vi "lv class tree.vi"() -> ()   [LabVIEW 2012]
uses:
  <vilib>/_script/All Supported PropertiesOrMethods TypeDefs/ASC_ArrayOfUniqueIDStringParentIDStringName.ctl
  <vilib>/_script/All Supported PropertiesOrMethods TypeDefs/ASC_UniqueIDStringParentIDStringName.ctl
panel:
  out "parent_children":cluster{i32[], string[], i32[], string[]}[](array[cluster])
  out "children":T1(array[cluster])
  out "sorted array 2":cluster{i32[], string[]}[](array[cluster])
  out "element 3":T2
  in  "element":string
  out "sorted array":T3(array[cluster])
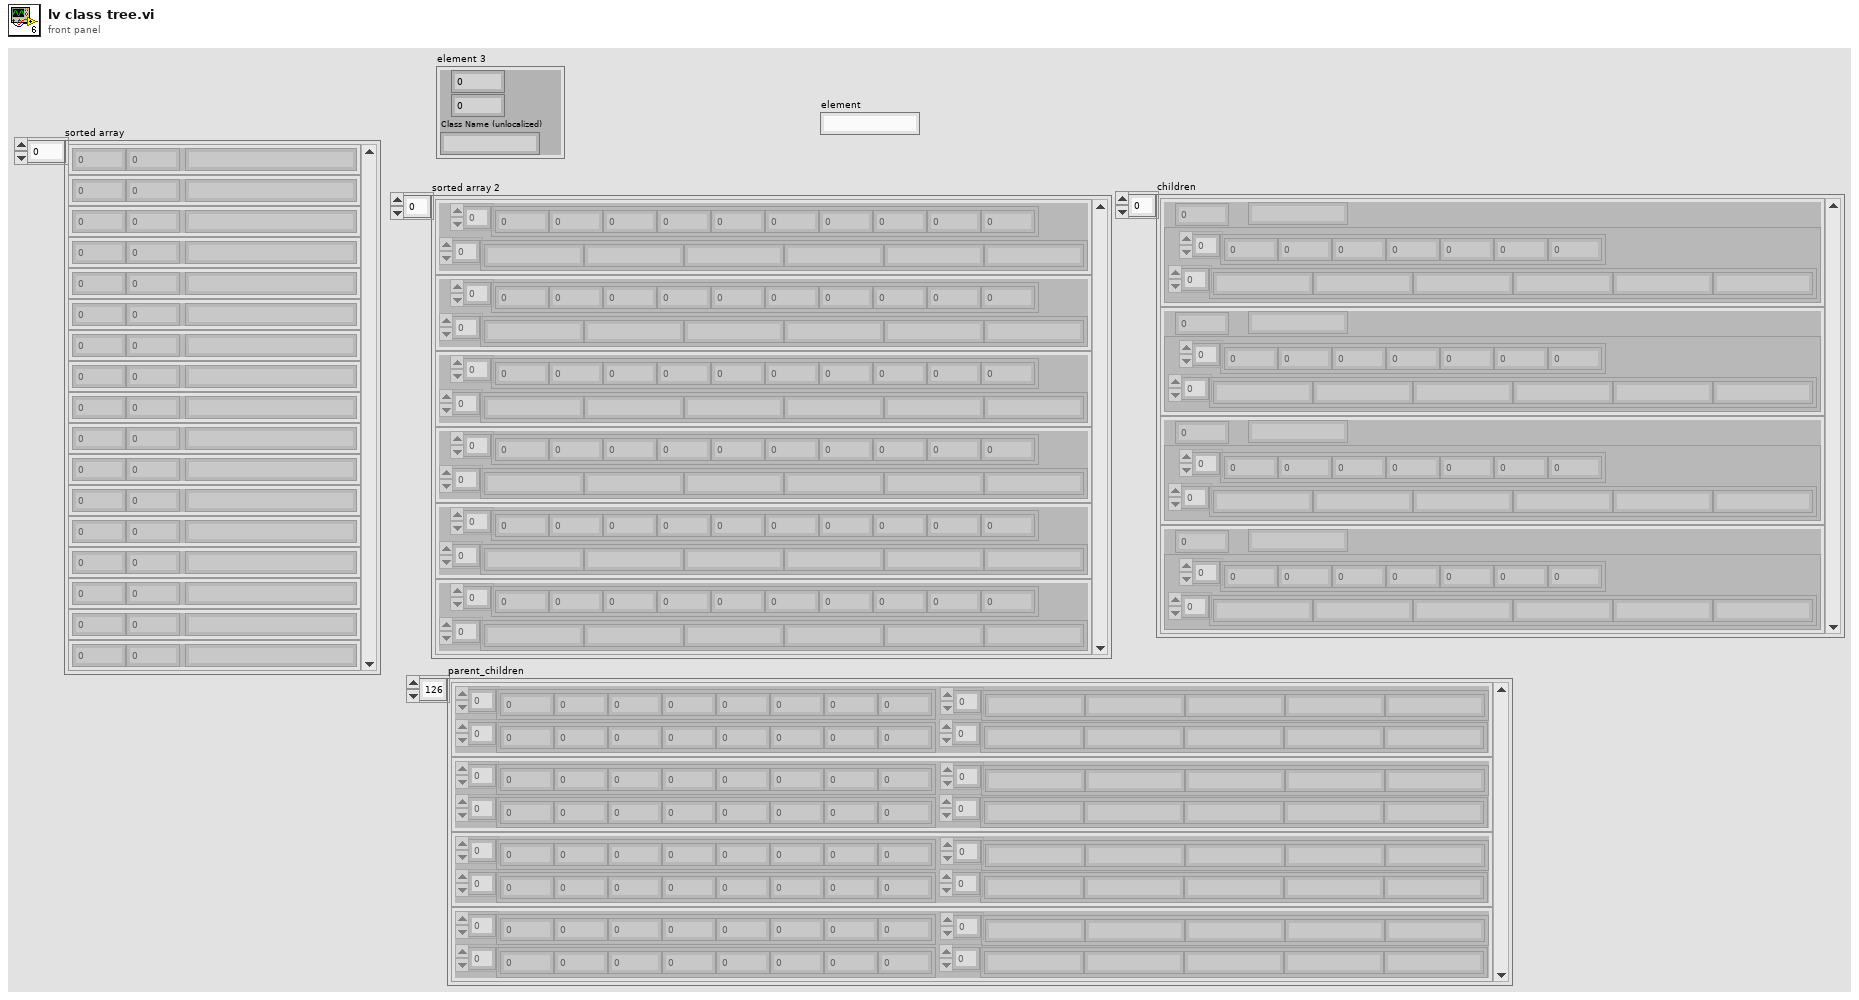
[diagram p1: front panel]
types:
  T1 = cluster{i32, cluster{i32[], string[]}, "Class Name (unlocalized)":string}[]
  T2 = cluster{i32, i32, "Class Name (unlocalized)":string}
  T3 = cluster{i32, i32, "Class Name (unlocalized)":string}[]
  T4 = typedef "ASC_ArrayOfUniqueIDStringParentIDStringName.ctl" = T5[]
  T5 = typedef "ASC_UniqueIDStringParentIDStringName.ctl" = cluster{"Unique ID string":string, "Parent ID string":string, "Class Name (unlocalized)":string, "Class Name (localized)":string}
  T6 = cluster{"Class Name (unlocalized)":string, i32, i32}
  T7 = cluster{"Class Name (unlocalized)":string, i32, i32}[]
  T8 = cluster{i32, cluster{i32[], string[]}, "Class Name (unlocalized)":string}
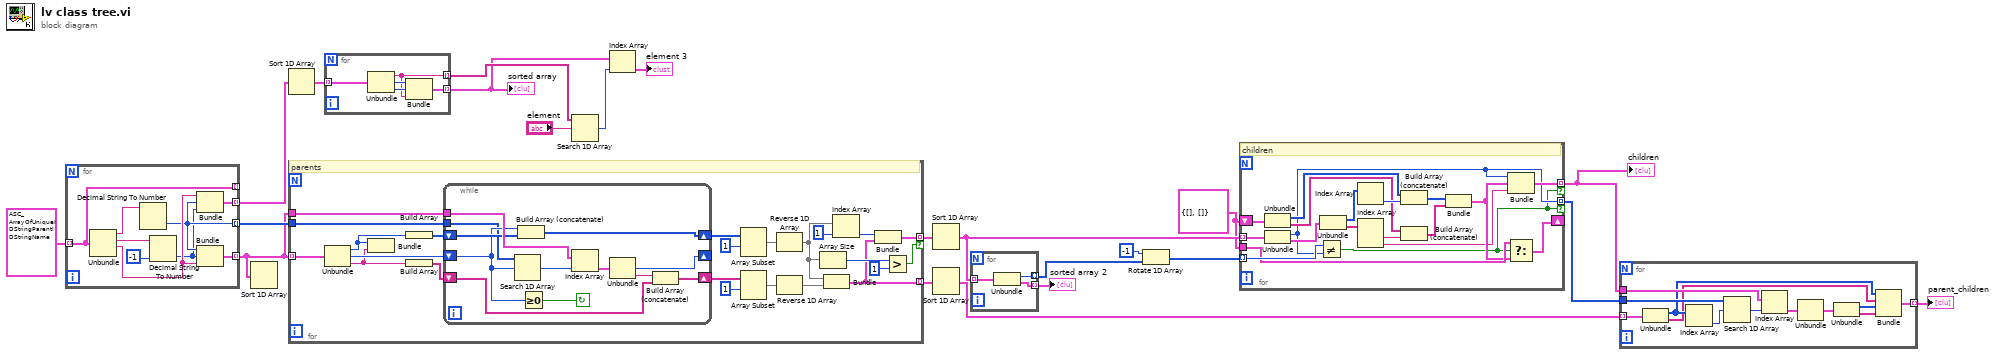
[diagram p0: block diagram]
diagram:
  w6 = cluster{i32[], string[]} {[], []} ("output cluster")
  n1 = for {
    tunnel: [w27] -> _ mode=indexing
    tunnel: [w28] -> w19 mode=indexing
    tunnel: [w25] -> w22 mode=indexing
    tunnel: T4 [{"Unique ID string"="3", "Parent ID string"="", "Class Name (unlocalized)"="Generic", "Class Name (localized)"="Generic"}, {"Unique ID string"="1", "Parent ID string"="", "Class Name (unlocalized)"="Application", "Class Name (localized)"="Application"}, {"Unique ID string"="2", "Parent ID string"="", "Class Name (unlocalized)"="VI", "Class Name (localized)"="VI"}, {"Unique ID string"="73", "Parent ID string"="", "Class Name (unlocalized)"="Project", "Class Name (localized)"="Project"}, {"Unique ID string"="74", "Parent ID string"="", "Class Name (unlocalized)"="ProjectItem", "Class Name (localized)"="ProjectItem"}, {"Unique ID string"="101", "Parent ID string"="2", "Class Name (unlocalized)"="PolymorphicVI", "Class Name (localized)"="PolymorphicVI"}, {"Unique ID string"="79", "Parent ID string"="2", "Class Name (unlocalized)"="FacadeVI", "Class Name (localized)"="FacadeVI"}, {"Unique ID string"="80", "Parent ID string"="74", "Class Name (unlocalized)"="Library", "Class Name (localized)"="Library"}, {"Unique ID string"="81", "Parent ID string"="", "Class Name (unlocalized)"="Variable", "Class Name (localized)"="Variable"}, {"Unique ID string"="82", "Parent ID string"="", "Class Name (unlocalized)"="TagSet", "Class Name (localized)"="TagSet"}, {"Unique ID string"="87", "Parent ID string"="2", "Class Name (unlocalized)"="MethodVI", "Class Name (localized)"="MethodVI"}, {"Unique ID string"="103", "Parent ID string"="80", "Class Name (unlocalized)"="XInterfaceLibrary", "Class Name (localized)"="XInterfaceLibrary"}, {"Unique ID string"="88", "Parent ID string"="103", "Class Name (unlocalized)"="XControlLibrary", "Class Name (localized)"="XControlLibrary"}, {"Unique ID string"="91", "Parent ID string"="", "Class Name (unlocalized)"="LVTarget", "Class Name (localized)"="LVTarget"}, {"Unique ID string"="93", "Parent ID string"="", "Class Name (unlocalized)"="Provider", "Class Name (localized)"="Provider"}, {"Unique ID string"="94", "Parent ID string"="", "Class Name (unlocalized)"="CopyOperation", "Class Name (localized)"="CopyOperation"}, {"Unique ID string"="95", "Parent ID string"="74", "Class Name (unlocalized)"="TargetItem", "Class Name (localized)"="TargetItem"}, {"Unique ID string"="96", "Parent ID string"="", "Class Name (unlocalized)"="ProjectItemType", "Class Name (localized)"="ProjectItemType"}, {"Unique ID string"="97", "Parent ID string"="", "Class Name (unlocalized)"="CopyItem", "Class Name (localized)"="CopyItem"}, {"Unique ID string"="98", "Parent ID string"="", "Class Name (unlocalized)"="CopyConflict", "Class Name (localized)"="CopyConflict"}, {"Unique ID string"="99", "Parent ID string"="", "Class Name (unlocalized)"="CopyExpert", "Class Name (localized)"="CopyExpert"}, {"Unique ID string"="123", "Parent ID string"="", "Class Name (unlocalized)"="Scene", "Class Name (localized)"="Scene"}, {"Unique ID string"="111", "Parent ID string"="123", "Class Name (unlocalized)"="SceneTexture", "Class Name (localized)"="SceneTexture"}, {"Unique ID string"="104", "Parent ID string"="123", "Class Name (unlocalized)"="SceneNode", "Class Name (localized)"="SceneNode"}, {"Unique ID string"="106", "Parent ID string"="104", "Class Name (unlocalized)"="SceneLight", "Class Name (localized)"="SceneLight"}, {"Unique ID string"="128", "Parent ID string"="123", "Class Name (unlocalized)"="SceneDrawable", "Class Name (localized)"="SceneDrawable"}, {"Unique ID string"="112", "Parent ID string"="128", "Class Name (unlocalized)"="SceneGeometry", "Class Name (localized)"="SceneGeometry"}, {"Unique ID string"="118", "Parent ID string"="112", "Class Name (unlocalized)"="SceneMesh", "Class Name (localized)"="SceneMesh"}, {"Unique ID string"="116", "Parent ID string"="112", "Class Name (unlocalized)"="SceneHeightField", "Class Name (localized)"="SceneHeightField"}, {"Unique ID string"="115", "Parent ID string"="112", "Class Name (unlocalized)"="SceneCylinder", "Class Name (localized)"="SceneCylinder"}, {"Unique ID string"="117", "Parent ID string"="112", "Class Name (unlocalized)"="SceneSphere", "Class Name (localized)"="SceneSphere"}, {"Unique ID string"="114", "Parent ID string"="112", "Class Name (unlocalized)"="SceneCone", "Class Name (localized)"="SceneCone"}, {"Unique ID string"="113", "Parent ID string"="112", "Class Name (unlocalized)"="SceneBox", "Class Name (localized)"="SceneBox"}, {"Unique ID string"="105", "Parent ID string"="104", "Class Name (unlocalized)"="SceneObject", "Class Name (localized)"="SceneObject"}, {"Unique ID string"="110", "Parent ID string"="104", "Class Name (unlocalized)"="SceneClipPlane", "Class Name (localized)"="SceneClipPlane"}, {"Unique ID string"="84", "Parent ID string"="123", "Class Name (unlocalized)"="SceneWindow", "Class Name (localized)"="SceneWindow"}, {"Unique ID string"="120", "Parent ID string"="74", "Class Name (unlocalized)"="PropertyFolder", "Class Name (localized)"="PropertyFolder"}, {"Unique ID string"="119", "Parent ID string"="120", "Class Name (unlocalized)"="XPropertyFolder", "Class Name (localized)"="XPropertyFolder"}, {"Unique ID string"="125", "Parent ID string"="74", "Class Name (unlocalized)"="LibraryData", "Class Name (localized)"="LibraryData"}, {"Unique ID string"="129", "Parent ID string"="128", "Class Name (unlocalized)"="SceneText", "Class Name (localized)"="SceneText"}, {"Unique ID string"="62", "Parent ID string"="2", "Class Name (unlocalized)"="SubsystemVI", "Class Name (localized)"="SubsystemVI"}, {"Unique ID string"="133", "Parent ID string"="", "Class Name (unlocalized)"="ProjectFilesViewItem", "Class Name (localized)"="ProjectFilesViewItem"}, {"Unique ID string"="134", "Parent ID string"="74", "Class Name (unlocalized)"="LVClassPropDefFolder", "Class Name (localized)"="LVClassPropDefFolder"}, {"Unique ID string"="36", "Parent ID string"="3", "Class Name (unlocalized)"="GObject", "Class Name (localized)"="GObject"}, {"Unique ID string"="37", "Parent ID string"="3", "Class Name (unlocalized)"="Plot", "Class Name (localized)"="Plot"}, {"Unique ID string"="38", "Parent ID string"="3", "Class Name (unlocalized)"="Cursor", "Class Name (localized)"="Cursor"}, {"Unique ID string"="4", "Parent ID string"="36", "Class Name (unlocalized)"="Decoration", "Class Name (localized)"="Decoration"}, {"Unique ID string"="5", "Parent ID string"="4", "Class Name (unlocalized)"="Text", "Class Name (localized)"="Text"}, {"Unique ID string"="39", "Parent ID string"="5", "Class Name (unlocalized)"="NumericText", "Class Name (localized)"="NumericText"}, {"Unique ID string"="40", "Parent ID string"="36", "Class Name (unlocalized)"="Scale", "Class Name (localized)"="Scale"}, {"Unique ID string"="41", "Parent ID string"="40", "Class Name (unlocalized)"="ColorScale", "Class Name (localized)"="ColorScale"}, {"Unique ID string"="42", "Parent ID string"="40", "Class Name (unlocalized)"="GraphScale", "Class Name (localized)"="GraphScale"}, {"Unique ID string"="43", "Parent ID string"="40", "Class Name (unlocalized)"="ColorGraphScale", "Class Name (localized)"="ColorGraphScale"}, {"Unique ID string"="6", "Parent ID string"="36", "Class Name (unlocalized)"="Control", "Class Name (localized)"="Control"}, {"Unique ID string"="7", "Parent ID string"="6", "Class Name (unlocalized)"="ColorBox", "Class Name (localized)"="ColorBox"}, {"Unique ID string"="8", "Parent ID string"="6", "Class Name (unlocalized)"="Boolean", "Class Name (localized)"="Boolean"}, {"Unique ID string"="9", "Parent ID string"="6", "Class Name (unlocalized)"="RefNum", "Class Name (localized)"="RefNum"}, {"Unique ID string"="44", "Parent ID string"="9", "Class Name (unlocalized)"="TypedRefNum", "Class Name (localized)"="TypedRefNum"}, {"Unique ID string"="10", "Parent ID string"="6", "Class Name (unlocalized)"="LVVariant", "Class Name (localized)"="LVVariant"}, {"Unique ID string"="11", "Parent ID string"="6", "Class Name (unlocalized)"="Path", "Class Name (localized)"="Path"}, {"Unique ID string"="12", "Parent ID string"="6", "Class Name (unlocalized)"="ListBox", "Class Name (localized)"="ListBox"}, {"Unique ID string"="13", "Parent ID string"="6", "Class Name (unlocalized)"="Table", "Class Name (localized)"="Table"}, {"Unique ID string"="14", "Parent ID string"="6", "Class Name (unlocalized)"="Array", "Class Name (localized)"="Array"}, {"Unique ID string"="15", "Parent ID string"="6", "Class Name (unlocalized)"="Picture", "Class Name (localized)"="Picture"}, {"Unique ID string"="16", "Parent ID string"="6", "Class Name (unlocalized)"="ActiveXContainer", "Class Name (localized)"="ActiveXContainer"}, {"Unique ID string"="17", "Parent ID string"="6", "Class Name (unlocalized)"="Numeric", "Class Name (localized)"="Numeric"}, {"Unique ID string"="18", "Parent ID string"="17", "Class Name (unlocalized)"="Digital", "Class Name (localized)"="Digital"}, {"Unique ID string"="19", "Parent ID string"="17", "Class Name (unlocalized)"="NamedNumeric", "Class Name (localized)"="NamedNumeric"}, {"Unique ID string"="35", "Parent ID string"="19", "Class Name (unlocalized)"="Enum", "Class Name (localized)"="Enum"}, {"Unique ID string"="34", "Parent ID string"="19", "Class Name (unlocalized)"="Ring", "Class Name (localized)"="Ring"}, {"Unique ID string"="20", "Parent ID string"="17", "Class Name (unlocalized)"="ColorRamp", "Class Name (localized)"="ColorRamp"}, {"Unique ID string"="33", "Parent ID string"="17", "Class Name (unlocalized)"="NumericWithScale", "Class Name (localized)"="NumericWithScale"}, {"Unique ID string"="21", "Parent ID string"="33", "Class Name (unlocalized)"="Slide", "Class Name (localized)"="Slide"}, {"Unique ID string"="32", "Parent ID string"="33", "Class Name (unlocalized)"="Knob", "Class Name (localized)"="Knob"}, {"Unique ID string"="22", "Parent ID string"="6", "Class Name (unlocalized)"="GraphChart", "Class Name (localized)"="GraphChart"}, {"Unique ID string"="23", "Parent ID string"="22", "Class Name (unlocalized)"="WaveformChart", "Class Name (localized)"="WaveformChart"}, {"Unique ID string"="24", "Parent ID string"="22", "Class Name (unlocalized)"="WaveformGraph", "Class Name (localized)"="WaveformGraph"}, {"Unique ID string"="25", "Parent ID string"="22", "Class Name (unlocalized)"="IntensityChart", "Class Name (localized)"="IntensityChart"}, {"Unique ID string"="26", "Parent ID string"="22", "Class Name (unlocalized)"="IntensityGraph", "Class Name (localized)"="IntensityGraph"}, {"Unique ID string"="27", "Parent ID string"="6", "Class Name (unlocalized)"="String", "Class Name (localized)"="String"}, {"Unique ID string"="28", "Parent ID string"="6", "Class Name (unlocalized)"="IOName", "Class Name (localized)"="IOName"}, {"Unique ID string"="29", "Parent ID string"="27", "Class Name (unlocalized)"="ComboBox", "Class Name (localized)"="ComboBox"}, {"Unique ID string"="30", "Parent ID string"="6", "Class Name (unlocalized)"="Cluster", "Class Name (localized)"="Cluster"}, {"Unique ID string"="31", "Parent ID string"="36", "Class Name (unlocalized)"="Panel", "Class Name (localized)"="Panel"}, {"Unique ID string"="46", "Parent ID string"="6", "Class Name (unlocalized)"="MulticolumnListbox", "Class Name (localized)"="MulticolumnListbox"}, {"Unique ID string"="47", "Parent ID string"="6", "Class Name (unlocalized)"="WaveformData", "Class Name (localized)"="WaveformData"}, {"Unique ID string"="48", "Parent ID string"="28", "Class Name (unlocalized)"="DSCTag", "Class Name (localized)"="DSCTag"}, {"Unique ID string"="49", "Parent ID string"="28", "Class Name (unlocalized)"="DAQChannelName", "Class Name (localized)"="DAQChannelName"}, {"Unique ID string"="50", "Parent ID string"="28", "Class Name (unlocalized)"="VISAResourceName", "Class Name (localized)"="VISAResourceName"}, {"Unique ID string"="51", "Parent ID string"="28", "Class Name (unlocalized)"="IVILogicalName", "Class Name (localized)"="IVILogicalName"}, {"Unique ID string"="52", "Parent ID string"="40", "Class Name (unlocalized)"="SlideScale", "Class Name (localized)"="SlideScale"}, {"Unique ID string"="53", "Parent ID string"="6", "Class Name (unlocalized)"="PageSelector", "Class Name (localized)"="PageSelector"}, {"Unique ID string"="54", "Parent ID string"="3", "Class Name (unlocalized)"="Page", "Class Name (localized)"="Page"}, {"Unique ID string"="55", "Parent ID string"="53", "Class Name (unlocalized)"="TabControl", "Class Name (localized)"="TabControl"}, {"Unique ID string"="56", "Parent ID string"="3", "Class Name (unlocalized)"="ConnectorPane", "Class Name (localized)"="ConnectorPane"}, {"Unique ID string"="57", "Parent ID string"="28", "Class Name (unlocalized)"="DAQmxName", "Class Name (localized)"="DAQmxName"}, {"Unique ID string"="59", "Parent ID string"="9", "Class Name (unlocalized)"="LVObjectRefNum", "Class Name (localized)"="LVObjectRefNum"}, {"Unique ID string"="58", "Parent ID string"="59", "Class Name (unlocalized)"="VIRefNum", "Class Name (localized)"="VIRefNum"}, {"Unique ID string"="60", "Parent ID string"="6", "Class Name (unlocalized)"="AbsTime", "Class Name (localized)"="AbsTime"}, {"Unique ID string"="61", "Parent ID string"="6", "Class Name (unlocalized)"="DigitalTable", "Class Name (localized)"="DigitalTable"}, {"Unique ID string"="66", "Parent ID string"="6", "Class Name (unlocalized)"="TreeControl", "Class Name (localized)"="TreeControl"}, {"Unique ID string"="67", "Parent ID string"="28", "Class Name (unlocalized)"="GenClassTagRef", "Class Name (localized)"="GenClassTagRef"}, {"Unique ID string"="68", "Parent ID string"="9", "Class Name (unlocalized)"="GenClassRef", "Class Name (localized)"="GenClassRef"}, {"Unique ID string"="65", "Parent ID string"="6", "Class Name (unlocalized)"="SubPanel", "Class Name (localized)"="SubPanel"}, {"Unique ID string"="69", "Parent ID string"="41", "Class Name (unlocalized)"="RotaryColorScale", "Class Name (localized)"="RotaryColorScale"}, {"Unique ID string"="70", "Parent ID string"="6", "Class Name (unlocalized)"="PlugInControl", "Class Name (localized)"="PlugInControl"}, {"Unique ID string"="71", "Parent ID string"="6", "Class Name (unlocalized)"="PlugInDDODummyContainer", "Class Name (localized)"="PlugInDDODummyContainer"}, {"Unique ID string"="122", "Parent ID string"="28", "Class Name (unlocalized)"="GenClassTagFlatRef", "Class Name (localized)"="GenClassTagFlatRef"}, {"Unique ID string"="72", "Parent ID string"="30", "Class Name (unlocalized)"="RadioButtonsControl", "Class Name (localized)"="RadioButtonsControl"}, {"Unique ID string"="75", "Parent ID string"="36", "Class Name (unlocalized)"="Pane", "Class Name (localized)"="Pane"}, {"Unique ID string"="77", "Parent ID string"="74", "Class Name (unlocalized)"="BuildSpecification", "Class Name (localized)"="BuildSpecification"}, {"Unique ID string"="78", "Parent ID string"="6", "Class Name (unlocalized)"="Pixmap", "Class Name (localized)"="Pixmap"}, {"Unique ID string"="83", "Parent ID string"="24", "Class Name (unlocalized)"="XYGraph", "Class Name (localized)"="XYGraph"}, {"Unique ID string"="76", "Parent ID string"="36", "Class Name (unlocalized)"="Splitter", "Class Name (localized)"="Splitter"}, {"Unique ID string"="85", "Parent ID string"="80", "Class Name (unlocalized)"="LVClassLibrary", "Class Name (localized)"="LVClassLibrary"}, {"Unique ID string"="89", "Parent ID string"="103", "Class Name (unlocalized)"="XNodeLibrary", "Class Name (localized)"="XNodeLibrary"}, {"Unique ID string"="90", "Parent ID string"="6", "Class Name (unlocalized)"="Scrollbar", "Class Name (localized)"="Scrollbar"}, {"Unique ID string"="92", "Parent ID string"="22", "Class Name (unlocalized)"="MixedSignalGraph", "Class Name (localized)"="MixedSignalGraph"}, {"Unique ID string"="100", "Parent ID string"="6", "Class Name (unlocalized)"="SceneGraphDisplay", "Class Name (localized)"="SceneGraphDisplay"}, {"Unique ID string"="102", "Parent ID string"="6", "Class Name (unlocalized)"="LabVIEWClassControl", "Class Name (localized)"="LabVIEWClassControl"}, {"Unique ID string"="121", "Parent ID string"="24", "Class Name (unlocalized)"="DigitalGraph", "Class Name (localized)"="DigitalGraph"}, {"Unique ID string"="126", "Parent ID string"="80", "Class Name (unlocalized)"="StatechartLibrary", "Class Name (localized)"="StatechartLibrary"}, {"Unique ID string"="127", "Parent ID string"="6", "Class Name (unlocalized)"="MixedCheckbox", "Class Name (localized)"="MixedCheckbox"}, {"Unique ID string"="130", "Parent ID string"="6", "Class Name (unlocalized)"="MultiSegmentPipe", "Class Name (localized)"="MultiSegmentPipe"}, {"Unique ID string"="131", "Parent ID string"="3", "Class Name (unlocalized)"="Bus", "Class Name (localized)"="Bus"}, {"Unique ID string"="132", "Parent ID string"="6", "Class Name (unlocalized)"="StubDDO", "Class Name (localized)"="StubDDO"}, {"Unique ID string"="135", "Parent ID string"="44", "Class Name (unlocalized)"="DataValRefNum", "Class Name (localized)"="DataValRefNum"}, {"Unique ID string"="16503", "Parent ID string"="36", "Class Name (unlocalized)"="AbstractDiagram", "Class Name (localized)"="AbstractDiagram"}, {"Unique ID string"="16384", "Parent ID string"="16503", "Class Name (unlocalized)"="Diagram", "Class Name (localized)"="Diagram"}, {"Unique ID string"="16423", "Parent ID string"="16384", "Class Name (unlocalized)"="TopLevelDiagram", "Class Name (localized)"="TopLevelDiagram"}, {"Unique ID string"="16385", "Parent ID string"="36", "Class Name (unlocalized)"="Terminal", "Class Name (localized)"="Terminal"}, {"Unique ID string"="16386", "Parent ID string"="36", "Class Name (unlocalized)"="Constant", "Class Name (localized)"="Constant"}, {"Unique ID string"="16387", "Parent ID string"="16386", "Class Name (unlocalized)"="PathConstant", "Class Name (localized)"="PathConstant"}, {"Unique ID string"="16388", "Parent ID string"="16386", "Class Name (unlocalized)"="ArrayConstant", "Class Name (localized)"="ArrayConstant"}, {"Unique ID string"="16389", "Parent ID string"="16386", "Class Name (unlocalized)"="NumericConstant", "Class Name (localized)"="NumericConstant"}, {"Unique ID string"="16390", "Parent ID string"="16389", "Class Name (unlocalized)"="DigitalNumericConstant", "Class Name (localized)"="DigitalNumericConstant"}, {"Unique ID string"="16391", "Parent ID string"="16389", "Class Name (unlocalized)"="NamedNumericConstant", "Class Name (localized)"="NamedNumericConstant"}, {"Unique ID string"="16424", "Parent ID string"="16391", "Class Name (unlocalized)"="RingConstant", "Class Name (localized)"="RingConstant"}, {"Unique ID string"="16425", "Parent ID string"="16391", "Class Name (unlocalized)"="EnumConstant", "Class Name (localized)"="EnumConstant"}, {"Unique ID string"="16392", "Parent ID string"="16386", "Class Name (unlocalized)"="StringConstant", "Class Name (localized)"="StringConstant"}, {"Unique ID string"="16393", "Parent ID string"="16386", "Class Name (unlocalized)"="ClusterConstant", "Class Name (localized)"="ClusterConstant"}, {"Unique ID string"="16394", "Parent ID string"="16386", "Class Name (unlocalized)"="FixedConstant", "Class Name (localized)"="FixedConstant"}, {"Unique ID string"="16422", "Parent ID string"="16386", "Class Name (unlocalized)"="BooleanConstant", "Class Name (localized)"="BooleanConstant"}, {"Unique ID string"="16395", "Parent ID string"="16385", "Class Name (unlocalized)"="ControlTerminal", "Class Name (localized)"="ControlTerminal"}, {"Unique ID string"="16396", "Parent ID string"="36", "Class Name (unlocalized)"="FormulaParameter", "Class Name (localized)"="FormulaParameter"}, {"Unique ID string"="16426", "Parent ID string"="36", "Class Name (unlocalized)"="Tunnel", "Class Name (localized)"="Tunnel"}, {"Unique ID string"="16427", "Parent ID string"="16426", "Class Name (unlocalized)"="LoopTunnel", "Class Name (localized)"="LoopTunnel"}, {"Unique ID string"="16399", "Parent ID string"="16426", "Class Name (unlocalized)"="RightShiftRegister", "Class Name (localized)"="RightShiftRegister"}, {"Unique ID string"="16428", "Parent ID string"="36", "Class Name (unlocalized)"="SequenceLocal", "Class Name (localized)"="SequenceLocal"}, {"Unique ID string"="16421", "Parent ID string"="36", "Class Name (unlocalized)"="Node", "Class Name (localized)"="Node"}, {"Unique ID string"="16397", "Parent ID string"="16421", "Class Name (unlocalized)"="Global", "Class Name (localized)"="Global"}, {"Unique ID string"="16398", "Parent ID string"="16421", "Class Name (unlocalized)"="Local", "Class Name (localized)"="Local"}, {"Unique ID string"="16400", "Parent ID string"="16421", "Class Name (unlocalized)"="Function", "Class Name (localized)"="Function"}, {"Unique ID string"="16429", "Parent ID string"="16400", "Class Name (unlocalized)"="Comparison", "Class Name (localized)"="Comparison"}, {"Unique ID string"="16430", "Parent ID string"="16400", "Class Name (unlocalized)"="ReadWriteFile", "Class Name (localized)"="ReadWriteFile"}, {"Unique ID string"="16431", "Parent ID string"="16400", "Class Name (unlocalized)"="TypeCast", "Class Name (localized)"="TypeCast"}, {"Unique ID string"="16432", "Parent ID string"="16400", "Class Name (unlocalized)"="FlattenUnflattenString", "Class Name (localized)"="FlattenUnflattenString"}, {"Unique ID string"="16433", "Parent ID string"="16400", "Class Name (unlocalized)"="GPIBReadWrite", "Class Name (localized)"="GPIBReadWrite"}, {"Unique ID string"="16401", "Parent ID string"="16421", "Class Name (unlocalized)"="SubVI", "Class Name (localized)"="SubVI"}, {"Unique ID string"="16402", "Parent ID string"="16421", "Class Name (unlocalized)"="CallByRef", "Class Name (localized)"="CallByRef"}, {"Unique ID string"="16403", "Parent ID string"="16421", "Class Name (unlocalized)"="UnitCast", "Class Name (localized)"="UnitCast"}, {"Unique ID string"="16404", "Parent ID string"="16421", "Class Name (unlocalized)"="Structure", "Class Name (localized)"="Structure"}, {"Unique ID string"="16405", "Parent ID string"="16404", "Class Name (unlocalized)"="Loop", "Class Name (localized)"="Loop"}, {"Unique ID string"="16434", "Parent ID string"="16405", "Class Name (unlocalized)"="ForLoop", "Class Name (localized)"="ForLoop"}, {"Unique ID string"="16435", "Parent ID string"="16405", "Class Name (unlocalized)"="WhileLoop", "Class Name (localized)"="WhileLoop"}, {"Unique ID string"="16406", "Parent ID string"="16404", "Class Name (unlocalized)"="MultiFrameStructure", "Class Name (localized)"="MultiFrameStructure"}, {"Unique ID string"="16407", "Parent ID string"="16406", "Class Name (unlocalized)"="Sequence", "Class Name (localized)"="Sequence"}, {"Unique ID string"="16408", "Parent ID string"="16406", "Class Name (unlocalized)"="CaseStructure", "Class Name (localized)"="CaseStructure"}, {"Unique ID string"="16409", "Parent ID string"="16421", "Class Name (unlocalized)"="Formula", "Class Name (localized)"="Formula"}, {"Unique ID string"="16436", "Parent ID string"="16409", "Class Name (unlocalized)"="ScriptNode", "Class Name (localized)"="ScriptNode"}, {"Unique ID string"="16437", "Parent ID string"="16400", "Class Name (unlocalized)"="ArrayToCluster", "Class Name (localized)"="ArrayToCluster"}, {"Unique ID string"="16410", "Parent ID string"="16421", "Class Name (unlocalized)"="GrowableFunction", "Class Name (localized)"="GrowableFunction"}, {"Unique ID string"="16411", "Parent ID string"="16410", "Class Name (unlocalized)"="BuildClusterArray", "Class Name (localized)"="BuildClusterArray"}, {"Unique ID string"="16412", "Parent ID string"="16410", "Class Name (unlocalized)"="CompoundArithmetic", "Class Name (localized)"="CompoundArithmetic"}, {"Unique ID string"="16413", "Parent ID string"="16410", "Class Name (unlocalized)"="IndexArray", "Class Name (localized)"="IndexArray"}, {"Unique ID string"="16416", "Parent ID string"="16410", "Class Name (unlocalized)"="CIN", "Class Name (localized)"="CIN"}, {"Unique ID string"="16417", "Parent ID string"="16410", "Class Name (unlocalized)"="CallLibrary", "Class Name (localized)"="CallLibrary"}, {"Unique ID string"="16438", "Parent ID string"="16410", "Class Name (unlocalized)"="FormatScanString", "Class Name (localized)"="FormatScanString"}, {"Unique ID string"="16418", "Parent ID string"="16410", "Class Name (unlocalized)"="ObjectFunction", "Class Name (localized)"="ObjectFunction"}, {"Unique ID string"="16419", "Parent ID string"="16418", "Class Name (unlocalized)"="Property", "Class Name (localized)"="Property"}, {"Unique ID string"="16420", "Parent ID string"="16418", "Class Name (unlocalized)"="Invoke", "Class Name (localized)"="Invoke"}, {"Unique ID string"="16439", "Parent ID string"="36", "Class Name (unlocalized)"="Wire", "Class Name (localized)"="Wire"}, {"Unique ID string"="16440", "Parent ID string"="3", "Class Name (unlocalized)"="Probe", "Class Name (localized)"="Probe"}, {"Unique ID string"="16441", "Parent ID string"="16385", "Class Name (unlocalized)"="InnerTerminal", "Class Name (localized)"="InnerTerminal"}, {"Unique ID string"="16442", "Parent ID string"="16426", "Class Name (unlocalized)"="LeftShiftRegister", "Class Name (localized)"="LeftShiftRegister"}, {"Unique ID string"="16443", "Parent ID string"="16401", "Class Name (unlocalized)"="PolymorphicSubVI", "Class Name (localized)"="PolymorphicSubVI"}, {"Unique ID string"="16444", "Parent ID string"="36", "Class Name (unlocalized)"="PropertyItem", "Class Name (localized)"="PropertyItem"}, {"Unique ID string"="16445", "Parent ID string"="16386", "Class Name (unlocalized)"="IONameConstant", "Class Name (localized)"="IONameConstant"}, {"Unique ID string"="16446", "Parent ID string"="16445", "Class Name (unlocalized)"="DSCTagConstant", "Class Name (localized)"="DSCTagConstant"}, {"Unique ID string"="16447", "Parent ID string"="16445", "Class Name (unlocalized)"="DAQChannelNameConstant", "Class Name (localized)"="DAQChannelNameConstant"}, {"Unique ID string"="16448", "Parent ID string"="16445", "Class Name (unlocalized)"="VISAResourceNameConstant", "Class Name (localized)"="VISAResourceNameConstant"}, {"Unique ID string"="16449", "Parent ID string"="16445", "Class Name (unlocalized)"="IVILogicalNameConstant", "Class Name (localized)"="IVILogicalNameConstant"}, {"Unique ID string"="16450", "Parent ID string"="16386", "Class Name (unlocalized)"="ColorBoxConstant", "Class Name (localized)"="ColorBoxConstant"}, {"Unique ID string"="16451", "Parent ID string"="16421", "Class Name (unlocalized)"="ControlReferenceConstant", "Class Name (localized)"="ControlReferenceConstant"}, {"Unique ID string"="16453", "Parent ID string"="16401", "Class Name (unlocalized)"="ConfNode", "Class Name (localized)"="ConfNode"}, {"Unique ID string"="16456", "Parent ID string"="16385", "Class Name (unlocalized)"="OuterTerminal", "Class Name (localized)"="OuterTerminal"}, {"Unique ID string"="16457", "Parent ID string"="16445", "Class Name (unlocalized)"="DAQmxNameConstant", "Class Name (localized)"="DAQmxNameConstant"}, {"Unique ID string"="16458", "Parent ID string"="16406", "Class Name (unlocalized)"="EventStructure", "Class Name (localized)"="EventStructure"}, {"Unique ID string"="16459", "Parent ID string"="36", "Class Name (unlocalized)"="FlatSequence", "Class Name (localized)"="FlatSequence"}, {"Unique ID string"="16460", "Parent ID string"="16445", "Class Name (unlocalized)"="GenClassTagRefConstant", "Class Name (localized)"="GenClassTagRefConstant"}, {"Unique ID string"="16461", "Parent ID string"="16386", "Class Name (unlocalized)"="AbsTimeConstant", "Class Name (localized)"="AbsTimeConstant"}, {"Unique ID string"="16462", "Parent ID string"="16407", "Class Name (unlocalized)"="ExternalNode", "Class Name (localized)"="ExternalNode"}, {"Unique ID string"="16466", "Parent ID string"="16392", "Class Name (unlocalized)"="ComboBoxConstant", "Class Name (localized)"="ComboBoxConstant"}, {"Unique ID string"="16463", "Parent ID string"="3", "Class Name (unlocalized)"="SubWizard", "Class Name (localized)"="SubWizard"}, {"Unique ID string"="16455", "Parent ID string"="16463", "Class Name (unlocalized)"="StateDiagramWizard", "Class Name (localized)"="StateDiagramWizard"}, {"Unique ID string"="16464", "Parent ID string"="16396", "Class Name (unlocalized)"="ScriptNodeParameter", "Class Name (localized)"="ScriptNodeParameter"}, {"Unique ID string"="16465", "Parent ID string"="16421", "Class Name (unlocalized)"="StaticVIReference", "Class Name (localized)"="StaticVIReference"}, {"Unique ID string"="16467", "Parent ID string"="16435", "Class Name (unlocalized)"="TimedLoop", "Class Name (localized)"="TimedLoop"}, {"Unique ID string"="16470", "Parent ID string"="16445", "Class Name (unlocalized)"="GenClassTagFlatRefConstant", "Class Name (localized)"="GenClassTagFlatRefConstant"}, {"Unique ID string"="16472", "Parent ID string"="16384", "Class Name (unlocalized)"="SimDiagram", "Class Name (localized)"="SimDiagram"}, {"Unique ID string"="16473", "Parent ID string"="16384", "Class Name (unlocalized)"="CompanionDiagram", "Class Name (localized)"="CompanionDiagram"}, {"Unique ID string"="16474", "Parent ID string"="16404", "Class Name (unlocalized)"="SimulationNode", "Class Name (localized)"="SimulationNode"}, {"Unique ID string"="16476", "Parent ID string"="16410", "Class Name (unlocalized)"="Bundler", "Class Name (localized)"="Bundler"}, {"Unique ID string"="16477", "Parent ID string"="16410", "Class Name (unlocalized)"="Unbundler", "Class Name (localized)"="Unbundler"}, {"Unique ID string"="16414", "Parent ID string"="16476", "Class Name (unlocalized)"="BuildArray", "Class Name (localized)"="BuildArray"}, {"Unique ID string"="16415", "Parent ID string"="16476", "Class Name (unlocalized)"="NamedBundler", "Class Name (localized)"="NamedBundler"}, {"Unique ID string"="16475", "Parent ID string"="36", "Class Name (unlocalized)"="SimulationDCO", "Class Name (localized)"="SimulationDCO"}, {"Unique ID string"="16478", "Parent ID string"="16477", "Class Name (unlocalized)"="NamedUnbundler", "Class Name (localized)"="NamedUnbundler"}, {"Unique ID string"="16479", "Parent ID string"="3", "Class Name (unlocalized)"="FlatSequenceFrame", "Class Name (localized)"="FlatSequenceFrame"}, {"Unique ID string"="16480", "Parent ID string"="36", "Class Name (unlocalized)"="FlatSequenceInnerTunnel", "Class Name (localized)"="FlatSequenceInnerTunnel"}, {"Unique ID string"="16481", "Parent ID string"="36", "Class Name (unlocalized)"="FlatSequenceOuterTunnel", "Class Name (localized)"="FlatSequenceOuterTunnel"}, {"Unique ID string"="16482", "Parent ID string"="16386", "Class Name (unlocalized)"="RefNumConstant", "Class Name (localized)"="RefNumConstant"}, {"Unique ID string"="16452", "Parent ID string"="16482", "Class Name (unlocalized)"="ClassSpecifierConstant", "Class Name (localized)"="ClassSpecifierConstant"}, {"Unique ID string"="16483", "Parent ID string"="16432", "Class Name (unlocalized)"="FlattenString", "Class Name (localized)"="FlattenString"}, {"Unique ID string"="16484", "Parent ID string"="36", "Class Name (unlocalized)"="PolymorphicVISelector", "Class Name (localized)"="PolymorphicVISelector"}, {"Unique ID string"="16485", "Parent ID string"="16421", "Class Name (unlocalized)"="XNode", "Class Name (localized)"="XNode"}, {"Unique ID string"="16486", "Parent ID string"="16525", "Class Name (unlocalized)"="SelectorTunnel", "Class Name (localized)"="SelectorTunnel"}, {"Unique ID string"="16487", "Parent ID string"="16406", "Class Name (unlocalized)"="DisableStructure", "Class Name (localized)"="DisableStructure"}, {"Unique ID string"="16491", "Parent ID string"="36", "Class Name (unlocalized)"="SynchronousDataFlowDCO", "Class Name (localized)"="SynchronousDataFlowDCO"}, {"Unique ID string"="16490", "Parent ID string"="16404", "Class Name (unlocalized)"="SynchronousDataFlowNode", "Class Name (localized)"="SynchronousDataFlowNode"}, {"Unique ID string"="16489", "Parent ID string"="16384", "Class Name (unlocalized)"="SDF Companion Diagram", "Class Name (localized)"="SDF Companion Diagram"}, {"Unique ID string"="16488", "Parent ID string"="16384", "Class Name (unlocalized)"="SDFDiagram", "Class Name (localized)"="SDFDiagram"}, {"Unique ID string"="16492", "Parent ID string"="16400", "Class Name (unlocalized)"="FileDialog", "Class Name (localized)"="FileDialog"}, {"Unique ID string"="16498", "Parent ID string"="16463", "Class Name (unlocalized)"="CodeWizard", "Class Name (localized)"="CodeWizard"}, {"Unique ID string"="16454", "Parent ID string"="3", "Class Name (unlocalized)"="MasterWizard", "Class Name (localized)"="MasterWizard"}, {"Unique ID string"="16494", "Parent ID string"="16479", "Class Name (unlocalized)"="TimeSequenceFrame", "Class Name (localized)"="TimeSequenceFrame"}, {"Unique ID string"="16495", "Parent ID string"="16459", "Class Name (unlocalized)"="TimeFlatSequence", "Class Name (localized)"="TimeFlatSequence"}, {"Unique ID string"="16496", "Parent ID string"="16404", "Class Name (unlocalized)"="TimedSequence", "Class Name (localized)"="TimedSequence"}, {"Unique ID string"="16493", "Parent ID string"="36", "Class Name (unlocalized)"="TimedStructDCO", "Class Name (localized)"="TimedStructDCO"}, {"Unique ID string"="16497", "Parent ID string"="16485", "Class Name (unlocalized)"="XDataNode", "Class Name (localized)"="XDataNode"}, {"Unique ID string"="16499", "Parent ID string"="16409", "Class Name (unlocalized)"="MathScriptNode", "Class Name (localized)"="MathScriptNode"}, {"Unique ID string"="16500", "Parent ID string"="16396", "Class Name (unlocalized)"="MathScriptNodeParameter", "Class Name (localized)"="MathScriptNodeParameter"}, {"Unique ID string"="16501", "Parent ID string"="16386", "Class Name (unlocalized)"="LabVIEWClassConstant", "Class Name (localized)"="LabVIEWClassConstant"}, {"Unique ID string"="16502", "Parent ID string"="16503", "Class Name (unlocalized)"="MathDiagram", "Class Name (localized)"="MathDiagram"}, {"Unique ID string"="16505", "Parent ID string"="16418", "Class Name (unlocalized)"="Constructor", "Class Name (localized)"="Constructor"}, {"Unique ID string"="16537", "Parent ID string"="16404", "Class Name (unlocalized)"="StatechartStructureNode", "Class Name (localized)"="StatechartStructureNode"}, {"Unique ID string"="16510", "Parent ID string"="16537", "Class Name (unlocalized)"="JoinNode", "Class Name (localized)"="JoinNode"}, {"Unique ID string"="16509", "Parent ID string"="16537", "Class Name (unlocalized)"="ForkNode", "Class Name (localized)"="ForkNode"}, {"Unique ID string"="16508", "Parent ID string"="16537", "Class Name (unlocalized)"="StateNode", "Class Name (localized)"="StateNode"}, {"Unique ID string"="16507", "Parent ID string"="16537", "Class Name (unlocalized)"="JunctionNode", "Class Name (localized)"="JunctionNode"}, {"Unique ID string"="16506", "Parent ID string"="16537", "Class Name (unlocalized)"="RegionNode", "Class Name (localized)"="RegionNode"}, {"Unique ID string"="16511", "Parent ID string"="16384", "Class Name (unlocalized)"="ScDiagram", "Class Name (localized)"="ScDiagram"}, {"Unique ID string"="16512", "Parent ID string"="16421", "Class Name (unlocalized)"="SharedVariableNode", "Class Name (localized)"="SharedVariableNode"}, {"Unique ID string"="16514", "Parent ID string"="16385", "Class Name (unlocalized)"="ParameterTerminal", "Class Name (localized)"="ParameterTerminal"}, {"Unique ID string"="16515", "Parent ID string"="16514", "Class Name (unlocalized)"="OverridableParameterTerminal", "Class Name (localized)"="OverridableParameterTerminal"}, {"Unique ID string"="16516", "Parent ID string"="16404", "Class Name (unlocalized)"="InPlaceElementStructure", "Class Name (localized)"="InPlaceElementStructure"}, {"Unique ID string"="16517", "Parent ID string"="16421", "Class Name (unlocalized)"="InPlaceBorderNode", "Class Name (localized)"="InPlaceBorderNode"}, {"Unique ID string"="16521", "Parent ID string"="16517", "Class Name (unlocalized)"="InPlaceElementNode", "Class Name (localized)"="InPlaceElementNode"}, {"Unique ID string"="16520", "Parent ID string"="16517", "Class Name (unlocalized)"="InPlaceVariantNode", "Class Name (localized)"="InPlaceVariantNode"}, {"Unique ID string"="16518", "Parent ID string"="16517", "Class Name (unlocalized)"="InPlaceArrayNode", "Class Name (localized)"="InPlaceArrayNode"}, {"Unique ID string"="16519", "Parent ID string"="16517", "Class Name (unlocalized)"="InPlaceClusterNode", "Class Name (localized)"="InPlaceClusterNode"}, {"Unique ID string"="16522", "Parent ID string"="16421", "Class Name (unlocalized)"="FeedbackNode", "Class Name (localized)"="FeedbackNode"}, {"Unique ID string"="16523", "Parent ID string"="16421", "Class Name (unlocalized)"="MathScriptCallByRef", "Class Name (localized)"="MathScriptCallByRef"}, {"Unique ID string"="16524", "Parent ID string"="16517", "Class Name (unlocalized)"="InPlaceDataValRefNode", "Class Name (localized)"="InPlaceDataValRefNode"}, {"Unique ID string"="16525", "Parent ID string"="16426", "Class Name (unlocalized)"="ConditionalTunnel", "Class Name (localized)"="ConditionalTunnel"}, {"Unique ID string"="16526", "Parent ID string"="16401", "Class Name (unlocalized)"="AbstractDynamicDispatch", "Class Name (localized)"="AbstractDynamicDispatch"}, {"Unique ID string"="16527", "Parent ID string"="16526", "Class Name (unlocalized)"="DynamicDispatchSubVI", "Class Name (localized)"="DynamicDispatchSubVI"}, {"Unique ID string"="16528", "Parent ID string"="16526", "Class Name (unlocalized)"="CallParentNode", "Class Name (localized)"="CallParentNode"}, {"Unique ID string"="16504", "Parent ID string"="16409", "Class Name (unlocalized)"="InlineCNode", "Class Name (localized)"="InlineCNode"}, {"Unique ID string"="16529", "Parent ID string"="16482", "Class Name (unlocalized)"="GenClassRefConst", "Class Name (localized)"="GenClassRefConst"}, {"Unique ID string"="16530", "Parent ID string"="16517", "Class Name (unlocalized)"="InPlaceArraySplitNode", "Class Name (localized)"="InPlaceArraySplitNode"}, {"Unique ID string"="16531", "Parent ID string"="16421", "Class Name (unlocalized)"="SharedVariableDynamicOpen", "Class Name (localized)"="SharedVariableDynamicOpen"}, {"Unique ID string"="16532", "Parent ID string"="16421", "Class Name (unlocalized)"="SharedVariableDynamicRead", "Class Name (localized)"="SharedVariableDynamicRead"}, {"Unique ID string"="16533", "Parent ID string"="16421", "Class Name (unlocalized)"="SharedVariableDynamicWrite", "Class Name (localized)"="SharedVariableDynamicWrite"}, {"Unique ID string"="16534", "Parent ID string"="16401", "Class Name (unlocalized)"="GenericSubVI", "Class Name (localized)"="GenericSubVI"}, {"Unique ID string"="16535", "Parent ID string"="16429", "Class Name (unlocalized)"="InRangeAndCoerce", "Class Name (localized)"="InRangeAndCoerce"}, {"Unique ID string"="16536", "Parent ID string"="16426", "Class Name (unlocalized)"="RegionTunnel", "Class Name (localized)"="RegionTunnel"}, {"Unique ID string"="16538", "Parent ID string"="16482", "Class Name (unlocalized)"="TypedRefNumConstant", "Class Name (localized)"="TypedRefNumConstant"}, {"Unique ID string"="16539", "Parent ID string"="16538", "Class Name (unlocalized)"="DataValRefNumConstant", "Class Name (localized)"="DataValRefNumConstant"}] ("AllTypes[]") -> [w27] mode=indexing
    tunnel: [w23] -> w20 mode=indexing
    n2 = Unbundle(w27) -> ("Unique ID string"=w31:string, "Parent ID string"=w30:string, "Class Name (unlocalized)"=w26:string)  [unwired: 1 out]
    n3 = Decimal String To Number(string=w31) -> (number=w25:i32)  [unwired: 2 in, 1 out]
    n4 = Decimal String To Number(string=w30, default (0L)=-1 ("default (0 I32)")) -> (number=w24:i32)  [unwired: 1 in, 1 out]
    n5 = Bundle("Class Name (unlocalized)"=w26, w25, w24) -> (w23:T6)  [unwired: 1 in]
    n6 = Bundle(w25, w24, "Class Name (unlocalized)"=w26) -> (w28:T2)  [unwired: 1 in]
  }
  n7 = Sort 1D Array(array=w19) -> ()  [unwired: 1 out]
  n8 = Sort 1D Array(array=w20) -> (sorted array=w18:T7)
  n9 = for {
    tunnel: w19 -> [w54] mode=indexing
    tunnel: w19 -> [w53]
    tunnel: [w32] -> w11 mode=indexing
    tunnel: w22 -> [w50]
    tunnel: [w34] -> w12 mode=indexing if=w33
    # "parents"
    n10 = Unbundle(w54) -> (w46:i32, w47:i32, "Class Name (unlocalized)"=w45:string)
    n11 = Bundle(w46, "Class Name (unlocalized)"=w45) -> ()  [unwired: 1 in, 1 out]
    n12 = Build Array(w46) -> (w51:i32[])
    n13 = Build Array(w45) -> (w52:string[])
    n14 = while {
      tunnel: w53 -> [w66]
      shift-right: [w64] -> w49
      shift-left: w52 -> [w63]
      shift-right: [w62] -> w43
      shift-left: w51 -> [w61]
      shift-right: [w56] -> _
      shift-left: w47 -> [w60]
      tunnel: w50 -> [w57]
      stop <- w59 continue-if-true
      n15 = Search 1D Array(1D array=w57, element=w60) -> (index of element=w58:i32)  [unwired: 1 in]
      n16 = Build Array (concatenate)(w60, w61) -> (w62:i32[])
      n17 = Greater Or Equal To 0?(x=w60) -> (x >= 0?=w59:bool)
      n18 = Index Array(array=w66, index=w58) -> (element=w65:T2)
      n19 = Unbundle(w65) -> (w56:i32, "Class Name (unlocalized)"=w55:string)  [unwired: 1 out]
      n20 = Build Array (concatenate)(w55, w63) -> (w64:string[])
    }
    n21 = Array Subset(array=w43, index=1) -> (w41:i32[])  [unwired: 1 in]
    n22 = Array Subset(array=w49, index=1) -> (w42:string[])  [unwired: 1 in]
    n23 = Reverse 1D Array(array=w41) -> (reversed array=w38:i32[])
    n24 = Reverse 1D Array(array=w42) -> (reversed array=w40:string[])
    n25 = Array Size(array=w38) -> (size(s)=w37:i32)
    n26 = Bundle(w38, w40) -> (w32:cluster{i32[], string[]})  [unwired: 1 in]
    n27 = Index Array(array=w38, index=1) -> (element=w35:i32)
    n28 = Bundle(w35, w32) -> (w34:cluster{i32, cluster{i32[], string[]}})  [unwired: 1 in]
    n29 = Greater?(x=w37, y=1) -> (0:w33:bool)
  }
  n30 = for {
    tunnel: w18 -> [w71] mode=indexing
    tunnel: [w68] -> w14 mode=indexing
    tunnel: [w67] -> w17 mode=indexing
    n31 = Unbundle(w71) -> ("Class Name (unlocalized)"=w67:string, w70:i32, w69:i32)
    n32 = Bundle(w70, w69, "Class Name (unlocalized)"=w67) -> (w68:T2)  [unwired: 1 in]
  }
  "sorted array" <- w14
  n33 = Search 1D Array(1D array=w17, element="element") -> (index of element=w15:i32)  [unwired: 1 in]
  n34 = Index Array(array=w14, index=w15) -> (element=→"element 3":T2)
  n35 = Sort 1D Array(array=w12) -> (sorted array=w10:cluster{i32, cluster{i32[], string[]}}[])
  n36 = Sort 1D Array(array=w11) -> (sorted array=w4:cluster{i32[], string[]}[])
  n37 = for {
    tunnel: w10 -> [w74] mode=indexing
    tunnel: [w73] -> w9 mode=indexing
    tunnel: [w72] -> w5 mode=indexing
    n38 = Unbundle(w74) -> (w73:i32, w72:cluster{i32[], string[]})
  }
  "sorted array 2" <- w5
  n39 = Rotate 1D Array(1:w9, 2:-1 ("n")) -> (0:w7:i32[])
  n40 = for {
    tunnel: w10 -> [w93] mode=indexing
    shift-right: [w80] -> _
    shift-left: w6 -> [w87]
    tunnel: w7 -> [w89] mode=indexing
    tunnel: w6 -> [w88]
    tunnel: [w78] -> w2 mode=indexing if=w75
    tunnel: [w76] -> w3 mode=indexing if=w75
    # "children"
    n41 = Unbundle(w87) -> (w86:i32[], w84:string[])
    n42 = Unbundle(w93) -> (w76:i32, w92:cluster{i32[], string[]})
    n43 = Not Equal?(x=w89, y=w76) -> (x != y?=w75:bool)
    n44 = Unbundle(w92) -> (w91:i32[], w90:string[])
    n45 = Index Array(array=w91) -> (element=w85:i32)  [unwired: 1 in]
    n46 = Index Array(array=w90) -> (element #1=w83:string, element #2=w77:string)  [unwired: 2 in]
    n47 = Build Array (concatenate)(w86, w85) -> (w82:i32[])
    n48 = Build Array (concatenate)(w84, w83) -> (w81:string[])
    n49 = Bundle(w82, w81) -> (w79:cluster{i32[], string[]})  [unwired: 1 in]
    n50 = Bundle(w76, w79, "Class Name (unlocalized)"=w77) -> (w78:T8)  [unwired: 1 in]
    n51 = Select(t=w88, s=w75, f=w79) -> (s? t:f=w80:cluster{i32[], string[]})
  }
  "children" <- w2
  n52 = for {
    tunnel: w4 -> [w105] mode=indexing
    tunnel: w3 -> [w104]
    tunnel: w2 -> [w101]
    tunnel: [w94] -> w1 mode=indexing
    n53 = Unbundle(w105) -> (w100:i32[], w97:string[])
    n54 = Index Array(array=w100) -> (element=w103:i32)  [unwired: 1 in]
    n55 = Search 1D Array(1D array=w104, element=w103) -> (index of element=w102:i32)  [unwired: 1 in]
    n56 = Index Array(array=w101, index=w102) -> (element=w99:T8)
    n57 = Unbundle(w99) -> (w98:cluster{i32[], string[]})  [unwired: 2 out]
    n58 = Unbundle(w98) -> (w96:i32[], w95:string[])
    n59 = Bundle(w100, w97, w96, w95) -> (w94:cluster{i32[], string[], i32[], string[]})  [unwired: 1 in]
  }
  "parent_children" <- w1
